vi "VisionTurnSmooth2.vi"(5 "Min Power":dbl, 7 "Target Range":dbl, 8 "Current Position":dbl, 9 "Target Position":dbl, 11 "Motor Power In":dbl) -> (0 "Done":bool, 2 "Right Motor Power":dbl, 3 "Left Motor Power":dbl)   [LabVIEW 2016]
panel:
  in  "Multiplier":dbl
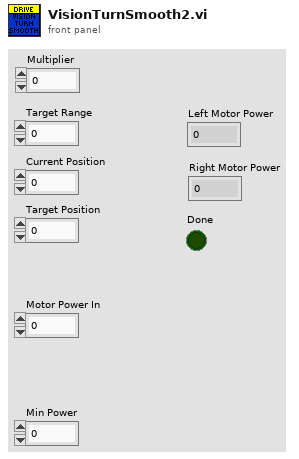
[diagram p1: front panel]
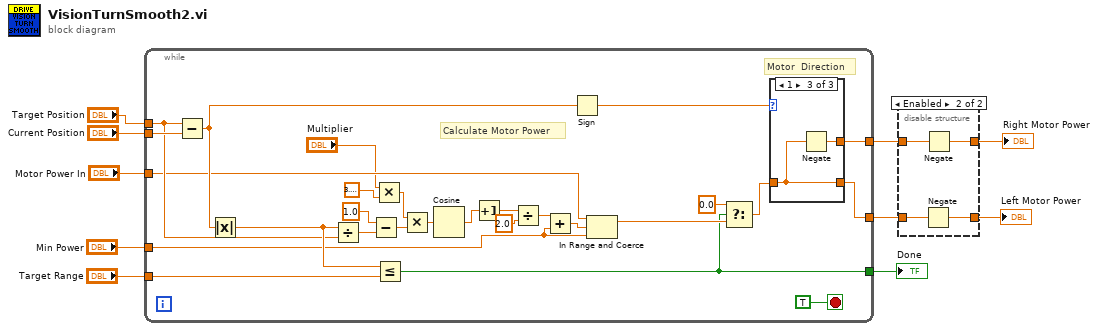
[diagram p0: block diagram]
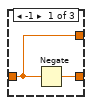
[diagram p3: hidden frame]
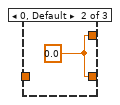
[diagram p4: hidden frame]
diagram:
  n1 = while {
    tunnel: [w30] -> w10
    tunnel: [w34] -> w4
    tunnel: [w33] -> w2
    tunnel: "Current Position" -> [w28]
    tunnel: "Target Position" -> [w26]
    tunnel: "Motor Power In" -> [w25]
    tunnel: "Min Power" -> [w14]
    tunnel: "Target Range" -> [w32]
    stop <- TRUE stop-if-true
    # "Motor  Direction"
    # "Calculate Motor Power"
    n2 = Subtract(x=w26, y=w28) -> (x-y=w36:dbl)
    n3 = Absolute Value(x=w36) -> (abs(x)=w27:dbl)
    n4 = Divide(x=w27, y=w26) -> (x/y=w23:dbl)
    n5 = Subtract(x=1.0, y=w23) -> (x-y=w21:dbl)
    n6 = Multiply(x="Multiplier", y=3.141592653589793) -> (x*y=w12:dbl)
    n7 = Less Or Equal?(x=w27, y=w32) -> (x <= y?=w30:bool)
    n8 = Multiply(x=w12, y=w21) -> (x*y=w20:dbl)
    n9 = Cosine(x=w20) -> (cos(x)=w17:dbl)
    n10 = Increment(x=w17) -> (x+1=w18:dbl)
    n11 = Divide(x=w18, y=2.0) -> (x/y=w16:dbl)
    n12 = Add(x=w16, y=w14) -> (x+y=w15:dbl)
    n13 = Sign(1:w36) -> (0:w35:dbl)
    n14 = In Range and Coerce(upper limit=w25, x=w15, lower limit=w14) -> (coerced(x)=w31:dbl)  [unwired: 1 out]
    n15 = Select(t=0.0, s=w30, f=w31) -> (s? t:f=w24:dbl)
    n16 = case shown="1" w35 {
      tunnel: [w39 w40 w41] -> w34
      tunnel: [w38 w40 w42] -> w33
      tunnel: w24 -> [w38 _ w41]
      frame -1 {
        n17 = Negate(x=w38) -> (-x=w39:dbl)
      }
      frame 0, Default {
        w40 = 0.0
      }
      frame 1 {
        n18 = Negate(x=w41) -> (-x=w42:dbl)
      }
    }
  }
  "Done" <- w10
  n19 = disable-structure shown="Enabled" {
    disable-tunnel: w4 -> [w44 w48]
    disable-tunnel: [w44 w47] -> w3
    disable-tunnel: w2 -> [w43 w46]
    disable-tunnel: [w43 w45] -> w1
    frame Disabled {
    }
    frame Enabled {
      n20 = Negate(x=w48) -> (-x=w47:dbl)
      n21 = Negate(x=w46) -> (-x=w45:dbl)
    }
  }
  "Left Motor Power" <- w3
  "Right Motor Power" <- w1
